vi "Dashboard Global Data.vi"() -> ()   [LabVIEW 2012]
doc: "This global VI can contain as many global variables as you need. Place a control on the panel, give it a good name. To read or write to it from a VI, drag the icon to the diagram of that VI. You can also drag from the project. Click on the node to change which global you access. You shouldn't have multiple locations writing to a global or it will cause a race-condition."
panel:
  in  "Test Logged":bool
  in  "Tele-Op Logged":bool
  in  "Auto Logged":bool
  in  "Robot Enabled":bool
  in  "Last String Robot":string
  in  "Robot Connected":bool
  out "LogFile":refnum<file>
  in  "LogArray":string[](array[string])
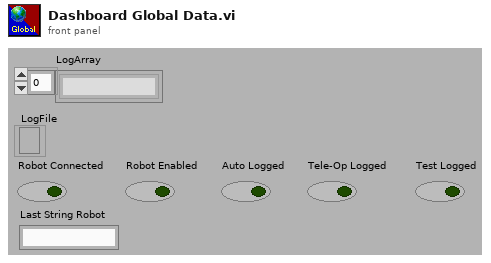
[diagram p1: front panel]
diagram:
